vi "IV_procedure_test.vi"() -> ()   [LabVIEW 2022 SP3]
uses:
  Supporting Files/IV_cluster_in.ctl
  <instrlib>/Keithley 648X Series/Keithley 648X Series.lvlib
panel:
  in  "Upper Measurement Range":u16(ring)=2 items=["20mA", "2mA", "200uA", "20uA", "2uA", "200nA", "20nA", "2nA"]
  out "IV curve":cluster{dbl[], dbl[]}(graph)
  in  "Forward/Reverse":u16(ring) items=["Reverse", "Forward"]
  in  "Input cluster":T1={"Vmin"=0.001, "Vmax"=0.001, "Step"=0.001, "milliseconds to wait"=10, "limit current [mA]"=0.001, "ms to ramp down"=10, "Stop"=FALSE} {"limit current [mA]" format="%#_13g"; "Step" format="%#_13g"; "Vmax" format="%#_13g"; "Vmin" format="%#_13g"}
  in  "Serial Configuration":T2={"Baud Rate"=9600, "Parity"=0, "Data Bits"=8, "Stop Bits"=10, "Flow Control"=0} {"Flow Control" items=["None", "XON/XOFF", "RTS/CTS", "XON/XOFF & RTS/CTS", "DTR/DSR", "XON/XOFF & DTR/DSR"]; "Stop Bits" items=["1.0"=10, "1.5"=15, "2.0"=20]; "Data Bits" items=["7"=7, "8"=8]; "Parity" items=["None", "Odd", "Even", "Mark", "Space"]; "Baud Rate" items=["300"=300, "600"=600, "1200"=1200, "2400"=2400, "4800"=4800, "9600"=9600, "19200"=19200]}
  in  "VISA resource name":refnum<visa-resource-name>
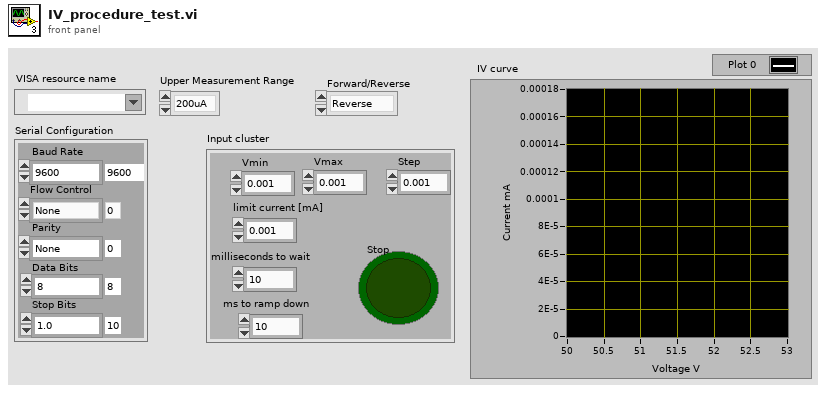
[diagram p1: front panel]
types:
  T1 = typedef "IV_cluster_in.ctl" = cluster{"Vmin":dbl, "Vmax":dbl, "Step":dbl, "milliseconds to wait":u32, "limit current [mA]":dbl, "ms to ramp down":u32, "Stop":bool}
  T2 = cluster{"Baud Rate":u32, "Parity":u16, "Data Bits":u16, "Stop Bits":u16, "Flow Control":u16}
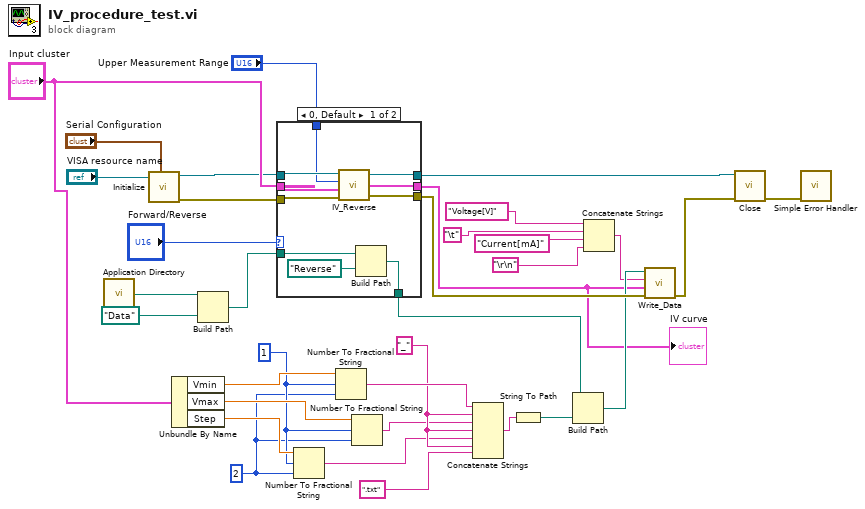
[diagram p0: block diagram]
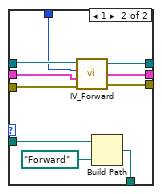
[diagram p2: hidden frame]
diagram:
  w11 = "_"
  w13 = 2
  w14 = 1
  n1 = call <vilib>:"Application Directory.vi"() -> ("Application Directory"=w31:path)
  n2 = call <instrlib>:"Initialize.vi"("Serial Configuration"="Serial Configuration", "VISA resource name"="VISA resource name") -> ("error out"=w2:errorcluster, "VISA resource name out"=w3:refnum<visa-resource-name>)  [unwired: 8 in]
  n3 = Unbundle By Name("Input cluster") -> ("Vmin"=w15:dbl, "Vmax"=w16:dbl, "Step"=w17:dbl)
  n4 = Build Path(base path=w31, name or relative path=path "Data") -> (appended path=w22:path)
  n5 = case shown="0, Default" "Forward/Reverse" {
    tunnel: w3 -> [w38 w46]
    tunnel: w2 -> [w36 w48]
    tunnel: [w39 w49] -> w32
    tunnel: [w40 w50] -> w4
    tunnel: "Input cluster" -> [w37 w47]
    tunnel: [w41 w51] -> w26
    tunnel: w22 -> [w43 w54]
    tunnel: [w44 w52] -> w20
    tunnel: "Upper Measurement Range" -> [w35 w45]
    frame 0, Default {
      n6 = call "IV_Reverse.vi"("error in (no error)"=w36, "Input cluster"=w37, "Upper Measurement Range"=w35, "VISA resource name in"=w38) -> ("error out"=w39:errorcluster, "IV cluster"=w40:cluster{dbl[], dbl[]}, "VISA resource name out"=w41:refnum<visa-resource-name>)
      n7 = Build Path(base path=w43, name or relative path=path "Reverse") -> (appended path=w44:path)
    }
    frame 1 {
      n8 = call "IV_Forward.vi"("error in (no error)"=w48, "Input cluster"=w47, "Upper Measurement Range"=w45, "VISA Keithley resource in"=w46) -> ("error out"=w49:errorcluster, "IV cluster"=w50:cluster{dbl[], dbl[]}, "VISA Keithley resource out"=w51:refnum<visa-resource-name>)
      n9 = Build Path(base path=w54, name or relative path=path "Forward") -> (appended path=w52:path)
    }
  }
  "IV curve" <- w4
  n10 = Number To Fractional String(number=w17, width (-)=w14, precision (6)=w13) -> (F-format string=w9:string)  [unwired: 1 in]
  n11 = Number To Fractional String(number=w15, width (-)=w14, precision (6)=w13) -> (F-format string=w12:string)  [unwired: 1 in]
  n12 = Number To Fractional String(number=w16, width (-)=w14, precision (6)=w13) -> (F-format string=w10:string)  [unwired: 1 in]
  n13 = Concatenate Strings(w12, w11, w10, w11, w9, w11, ".txt") -> (w29:string)
  n14 = String To Path(string=w29) -> (path=w28:path)
  n15 = Build Path(base path=w20, name or relative path=w28) -> (appended path=w27:path)
  n16 = Concatenate Strings("Voltage[V]", "\t", "Current[mA]", "\r\n") -> (w18:string)
  n17 = call "Write_Data.vi"("error in"=w32, "Data cluster in"=w4, "Header"=w18, "file path"=w27) -> ("error out"=w25:errorcluster)  [unwired: 3 in]
  n18 = call <instrlib>:"Close.vi"("error in (no error)"=w25, "VISA resource name"=w26) -> ("error out"=w24:errorcluster)  [unwired: 9 in]
  n19 = call <vilib>:"Simple Error Handler.vi"("error in (no error)"=w24) -> ()  [unwired: 4 in, 5 out]
